vi "ellipse fit data.vi"(7 "samples":i32, 8 "y0":dbl, 9 "x0":dbl, 10 "b":dbl, 11 "a":dbl) -> (2 "Y":dbl[](array[numeric]), 3 "X":dbl[](array[numeric]))   [LabVIEW 2023]
doc: "Ellipse fit data"
uses:
  <vilib>/Analysis/1siggen.llb/Ramp Pattern by Samples.vi
  <vilib>/Analysis/NI_AALBase.lvlib
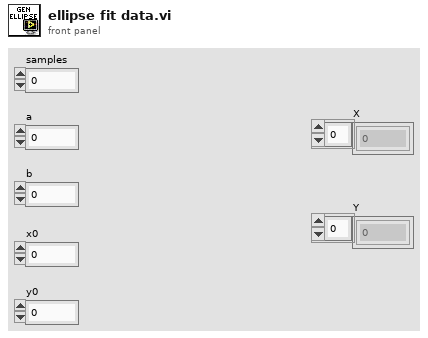
[diagram p1: front panel]
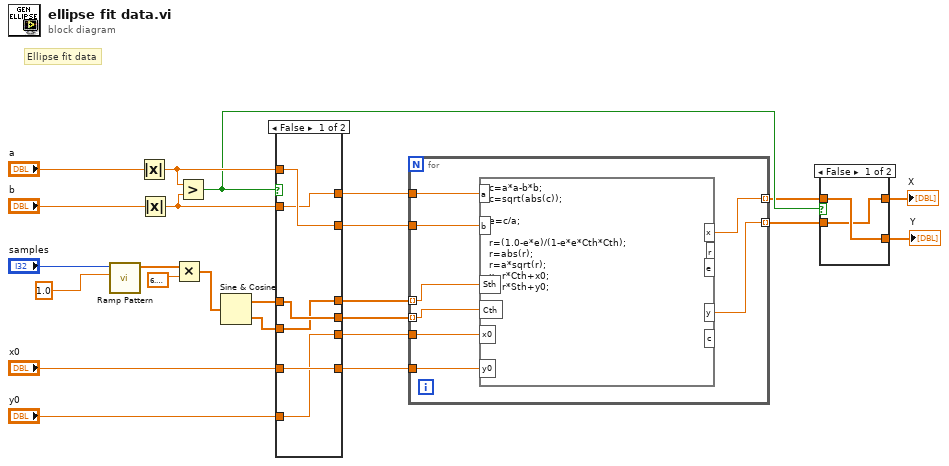
[diagram p0: block diagram]
diagram:
  # "Ellipse fit data"
  n1 = call-poly <vilib>:"Ramp Pattern.vi"("end"=1.0, "samples"="samples") -> ("Ramp Pattern"=w22:dbl[])  [unwired: 8 in, 1 out]
  n2 = Absolute Value(x="a") -> (abs(x)=w19:dbl)
  n3 = Absolute Value(x="b") -> (abs(x)=w18:dbl)
  n4 = Multiply(x=w22, y=6.283185307179586) -> (x*y=w14:dbl[])
  n5 = Greater?(x=w19, y=w18) -> (0:w8:bool)
  n6 = Sine & Cosine(0:w14) -> (1:w13:dbl[], 2:w12:dbl[])
  n7 = case shown="False" w8 {
    tunnel: w19 -> [w30 w36]
    tunnel: w18 -> [w29 w35]
    tunnel: [w29 w36] -> w17
    tunnel: [w30 w35] -> w16
    tunnel: w13 -> [w28 w34]
    tunnel: w12 -> [w27 w33]
    tunnel: [w27 w34] -> w11
    tunnel: [w28 w33] -> w10
    tunnel: "x0" -> [w26 w32]
    tunnel: "y0" -> [w25 w31]
    tunnel: [w25 w32] -> w2
    tunnel: [w26 w31] -> w1
    frame False {
    }
    frame True {
    }
  }
  n8 = for {
    tunnel: w17 -> [w44]
    tunnel: w16 -> [w43]
    tunnel: w2 -> [w42]
    tunnel: w1 -> [w41]
    tunnel: [w40] -> w7 mode=indexing
    tunnel: [w39] -> w9 mode=indexing
    tunnel: w11 -> [w38] mode=indexing
    tunnel: w10 -> [w37] mode=indexing
    n9 = formula code="c=a*a-b*b;\nc=sqrt(abs(c));\n\ne=c/a;\n\nr=(1.0-e*e)/(1-e*e*Cth*Cth);\nr=abs(r);\nr=a*sqrt(r);\nx=r*Cth+x0;\ny=r*Sth+y0;"("a"=w44, "b"=w43, "Sth"=w38, "x0"=w42, "y0"=w41, "Cth"=w37) -> ("x"=w40:dbl, "y"=w39:dbl)  [unwired: 3 out]
  }
  n10 = case shown="False" w8 {
    tunnel: w9 -> [w45 w48]
    tunnel: [w46 w48] -> w5
    tunnel: w7 -> [w46 w47]
    tunnel: [w45 w47] -> w6
    frame False {
    }
    frame True {
    }
  }
  "Y" <- w5
  "X" <- w6
